vi "control loop.vi"(6 "dt [s]":dbl, 8 "error in (no error)":errorcluster, 9 "Frequncey [Hz]":u16(slide)=1 max=10 step=1 scale=0.0..10.0, 10 "Reference":dbl(slide)=65.0 min=65.0 max=750.0 scale=0.0..500.0, 11 "controller in":refnum<class "controller.lvclass">) -> (0 "error out":errorcluster, 1 "input":dbl, 2 "State":dbl, 3 "controller out":refnum<class "controller.lvclass">)   [LabVIEW 2025, in "controller.lvclass"]
uses:
  controller.lvclass
  controller.lvclass/controller.ctl
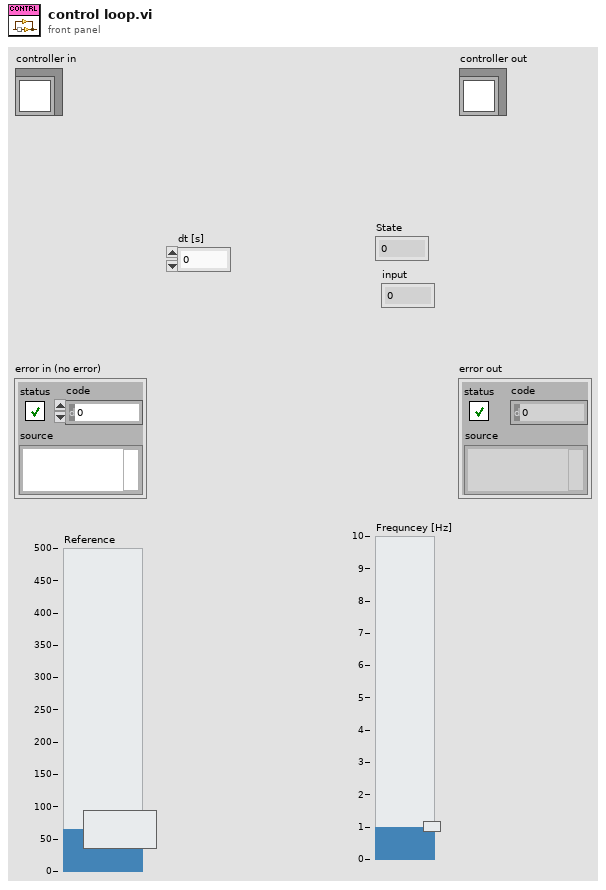
[diagram p1: front panel]
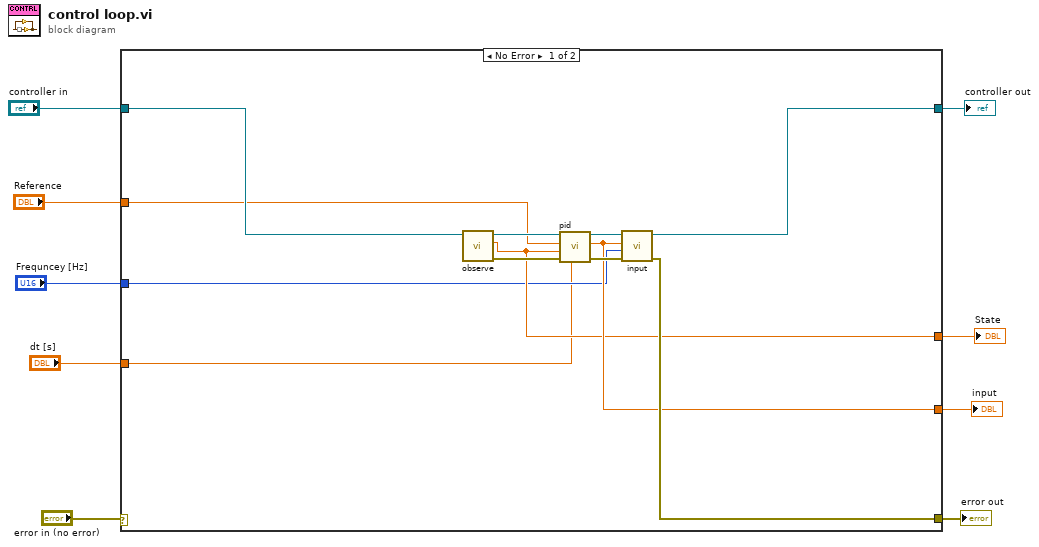
[diagram p0: block diagram]
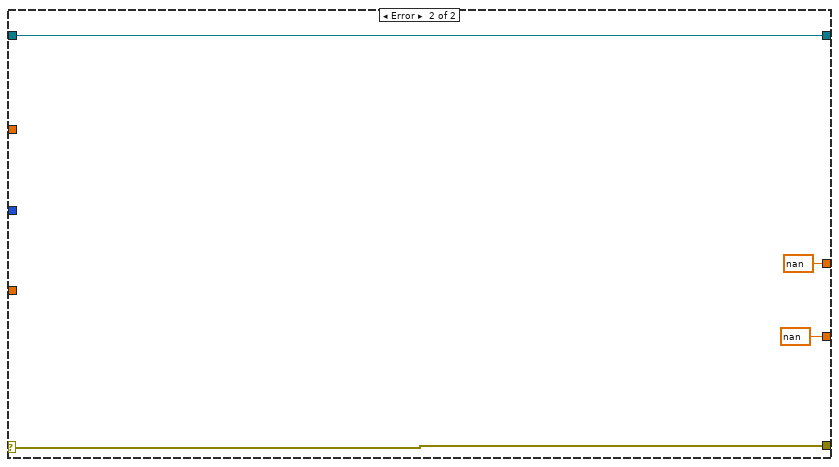
[diagram p2: hidden frame]
diagram:
  n1 = case shown="No Error" "error in (no error)" {
    selector: "error in (no error)" -> [_ w25]
    tunnel: [w16 w25] -> w8
    tunnel: [w15 w24] -> w6
    tunnel: "controller in" -> [w21 w24]
    tunnel: [w14 nan ("State")] -> w5
    tunnel: [w13 nan ("State")] -> w4
    tunnel: "Reference" -> [w12 _]
    tunnel: "Frequncey [Hz]" -> [w11 _]
    tunnel: "dt [s]" -> [w10 _]
    frame No Error {
      n2 = call-dynamic "observe.vi"("controller in"=w21) -> ("error out"=w17:errorcluster, "State"=w13:dbl, "controller out"=w18:refnum<class "controller.lvclass">)  [unwired: 8 in]
      n3 = call-dynamic "pid.vi"("dt [s]"=w10, "error in (no error)"=w17, "State"=w13, "Reference"=w12, "controller in"=w18) -> ("error out"=w19:errorcluster, "input"=w14:dbl, "controller out"=w20:refnum<class "controller.lvclass">)  [unwired: 4 in]
      n4 = call-dynamic "input.vi"("error in (no error)"=w19, "Frequncey [Hz]"=w11, "Duty Cycle [%]"=w14, "controller in"=w20) -> ("error out"=w16:errorcluster, "controller out"=w15:refnum<class "controller.lvclass">)  [unwired: 6 in]
    }
    frame Error {
    }
  }
  "error out" <- w8
  "controller out" <- w6
  "input" <- w5
  "State" <- w4
